vi "ADS Byte Stream Writer.vi"(8 "error in (no error)":errorcluster, 9 "Byte Stream In":u8[](array[numeric]), 11 "TwinCAT ADS in":refnum<class "TwinCAT ADS.lvclass">) -> (0 "error out":errorcluster, 1 "Byte Stream Out":u8[](array[numeric]), 2 ".NET AdsStream":refnum<k24>, 3 "TwinCAT ADS out":refnum<class "TwinCAT ADS.lvclass">)   [LabVIEW 2018, in "TwinCAT ADS.lvclass"]
uses:
  TwinCAT ADS.lvclass
  TwinCAT.Ads
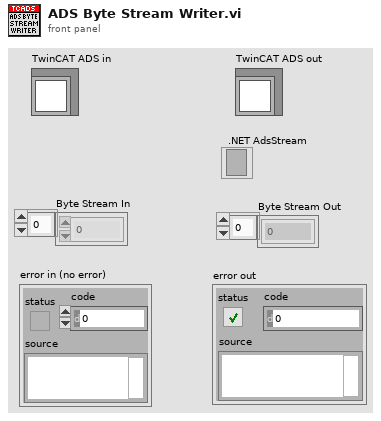
[diagram p1: front panel]
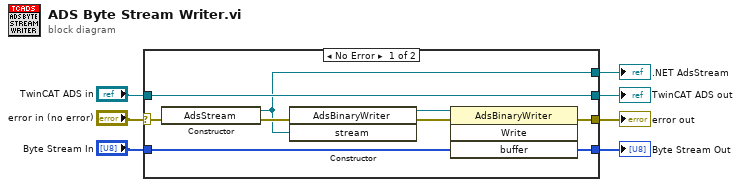
[diagram p0: block diagram]
diagram:
  n1 = case shown="No Error" "error in (no error)" {
    selector: "error in (no error)" -> [w12 w18]
    tunnel: [w9 w18] -> w7
    tunnel: "TwinCAT ADS in" -> [w11 w19]
    tunnel: [w11 w19] -> w5
    tunnel: "Byte Stream In" -> [w13 w17]
    tunnel: [w10 _] -> w2
    tunnel: [w8 w17] -> w1
    frame No Error {
      n2 = constructor class="AdsStream"(error in=w12) -> (reference out=w10:refnum<k24>, error out=w16:errorcluster)  [unwired: 2 in, 1 out]
      n3 = constructor class="AdsBinaryWriter"(error in=w16, "stream"=w10) -> (reference out=w14:refnum<k24>, error out=w15:errorcluster)  [unwired: 2 in, 2 out]
      n4 = invoke class="AdsBinaryWriter" method="Write"(reference=w14, error in=w15, "buffer"=w13) -> (error out=w9:errorcluster, "buffer"=w8:u8[])  [unwired: 1 in, 2 out]
    }
    frame Error {
    }
  }
  "error out" <- w7
  "TwinCAT ADS out" <- w5
  ".NET AdsStream" <- w2
  "Byte Stream Out" <- w1
